vi "IV2-LCRZ.vi"(0 "Voltage In":cdb=-0.04516796338063459+0.012130821220646867i format="%#_4p", 1 "Test Frequency":dbl=25000.0, 5 "Current In":cdb=0.0013952524174977166+0.030636391761552667i format="%#_4p", 12 "LCR Params":T2={"Rg_Vmon"=5000.0, "Rg_Imon"=5000.0, "ESL_Cal"=2.95e-07, "ESR_Cal"=0.0, "Cp_Cal"=0.0, "Rp_Cal"=1000000000.0, "Use Open/Short\nCompensation"=TRUE, "R_Shunt"=100.0}) -> (4 "Impedance (Mag)":dbl=0.0009831918388061723 format="%#_3p", 6 "Impedance (Phase)":dbl=169.4760326381836 format="%#_3p", 8 "Ls":dbl=9.665874386883538e-10 format="%#_3p", 10 "Cs":dbl=-0.029973703968004497 format="%#_3p", 14 "Impedance cluster":T3={"|Z|"=0.0009831918388061723, "Phase(Z)"=169.4760326381836, "Re(Z)"=-0.000966653166475792, "Imag(Z)"=0.00017957685718763175, "Ls"=9.665874386883538e-10, "Cs"=-0.029973703968004497, "Rp"=0.0, "Cp"=0.0}, 15 "Real (Z)":dbl=-0.000966653166475792 format="%#_3p")   [LabVIEW 2020]
panel:
  out "Z":cdb
  out "Y":cdb
  in  "Cal Cluster":T1={"ESL_Cal"=2e-07, "ESR_Cal"=0.0, "Cp_Cal"=0.0, "Rp_Cal"=1000000000.0}
  out "Current Phase\nDeg":dbl=87.39241896335173
  out "Z Phase (Pre)":dbl=77.5743267290552
  out "Z Mag (pre-correction)":dbl=152.4989366461181
  out "VGain":dbl=11.0 format="%#_3p"
  out "Detected Current\n(Measured Signal \nmagnitude)":dbl=0.030668146821675832 format="%#_3p"
  out "I_Gain":dbl=11.0 format="%#_3p"
  out "Imag(Z)":dbl=0.00017957685718763175 format="%#_3p"
  out "Voltage (mag)":dbl=0.004251690708375082 format="%#_3p"
  out "Current  (Amps)":dbl=2.7880133474250757e-05 format="%#_3p"
  out "Voltage Phase\n (deg)":dbl=164.96674569240693 format="%.2p"
  out "Detected Voltage\n(Measured Signal\nMagnitude":dbl=0.0467685977921259 format="%.2p"
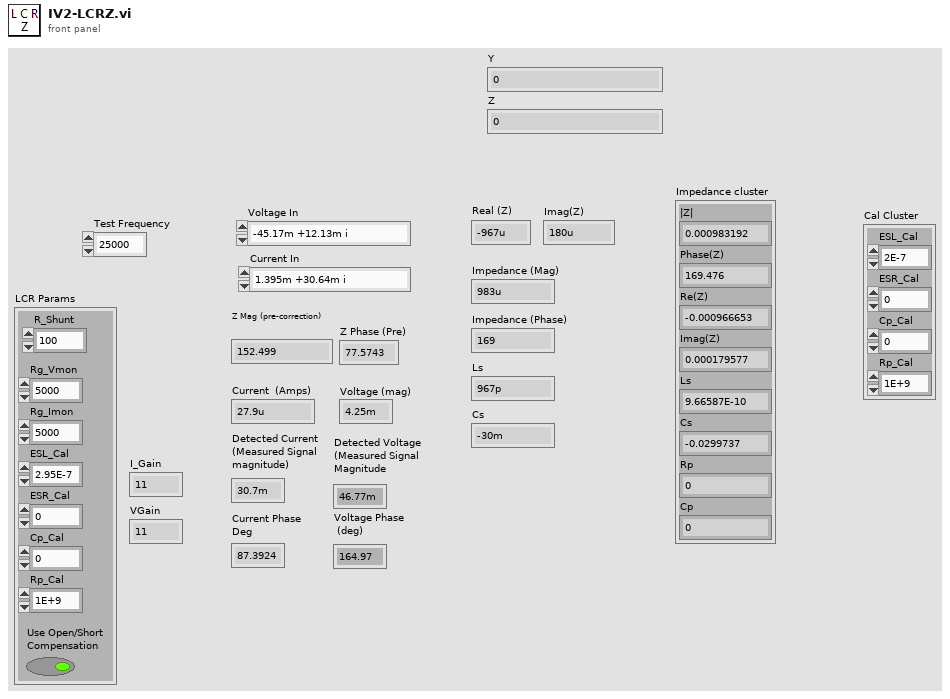
[diagram p1: front panel]
types:
  T1 = cluster{"ESL_Cal":dbl, "ESR_Cal":dbl, "Cp_Cal":dbl, "Rp_Cal":dbl}
  T2 = cluster{"Rg_Vmon":dbl, "Rg_Imon":dbl, "ESL_Cal":dbl, "ESR_Cal":dbl, "Cp_Cal":dbl, "Rp_Cal":dbl, "Use Open/Short\nCompensation":bool, "R_Shunt":dbl}
  T3 = cluster{"|Z|":dbl, "Phase(Z)":dbl, "Re(Z)":dbl, "Imag(Z)":dbl, "Ls":dbl, "Cs":dbl, "Rp":dbl, "Cp":dbl}
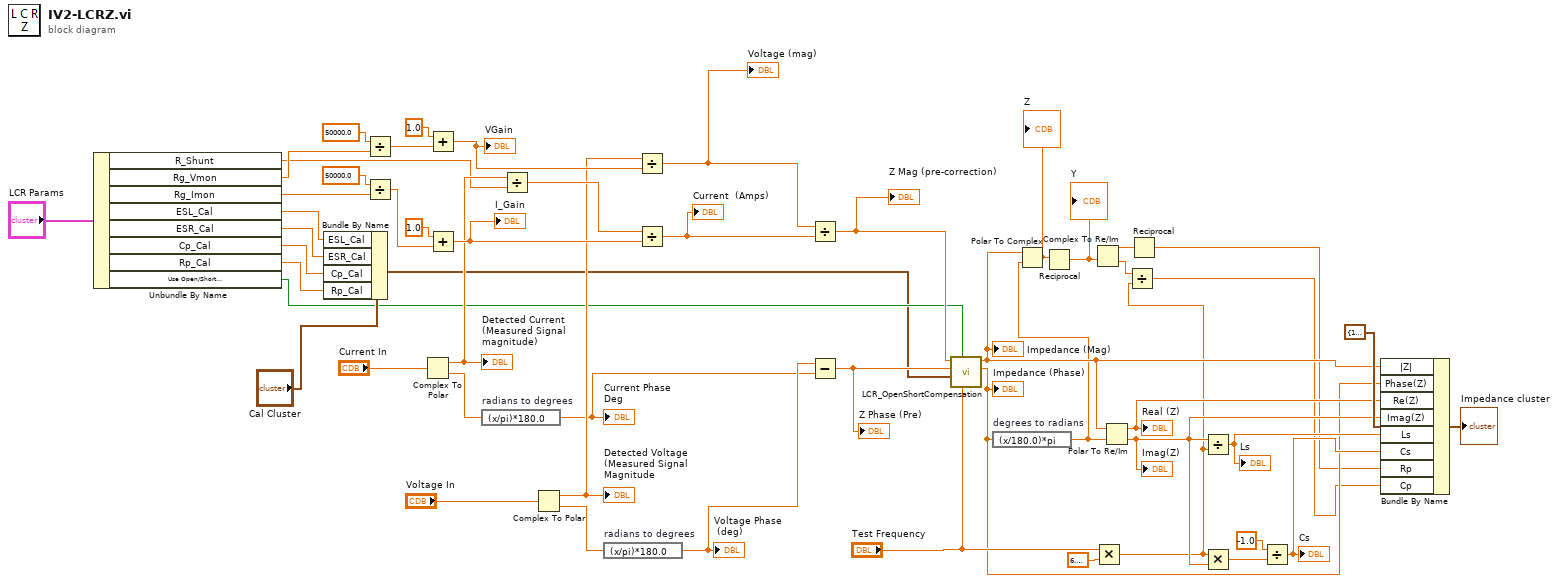
[diagram p0: block diagram]
diagram:
  n1 = Unbundle By Name("LCR Params") -> ("R_Shunt"=w12:dbl, "Rg_Vmon"=w14:dbl, "Rg_Imon"=w15:dbl, "ESL_Cal"=w19:dbl, "ESR_Cal"=w18:dbl, "Cp_Cal"=w17:dbl, "Rp_Cal"=w16:dbl, "Use Open/Short\nCompensation"=w13:bool)
  n2 = Bundle By Name(cluster="Cal Cluster", "ESL_Cal"=w19, "ESR_Cal"=w18, "Cp_Cal"=w17, "Rp_Cal"=w16) -> (w11:T1)
  n3 = Divide(x=50000.0, y=w14) -> (x/y=w44:dbl)
  n4 = Divide(x=50000.0, y=w15) -> (x/y=w48:dbl)
  n5 = Complex To Polar(r * e^(i*theta)="Current In") -> (r=w36:dbl, theta=w31:dbl)
  "Detected Current\n(Measured Signal \nmagnitude)" <- w36
  n6 = Add(x=1.0, y=w44) -> (x+y=w41:dbl)
  "VGain" <- w41
  n7 = Add(x=1.0, y=w48) -> (x+y=w46:dbl)
  "I_Gain" <- w46
  n8 = expression code="(x/pi)*180.0" "radians to degrees"(w31) -> (w30:dbl)
  "Current Phase\nDeg" <- w30
  n9 = Divide(x=w36, y=w12) -> (x/y=w47:dbl)
  n10 = Complex To Polar(r * e^(i*theta)="Voltage In") -> (r=w37:dbl, theta=w33:dbl)
  "Detected Voltage\n(Measured Signal\nMagnitude" <- w37
  n11 = expression code="(x/pi)*180.0" "radians to degrees"(w33) -> (w32:dbl)
  "Voltage Phase\n (deg)" <- w32
  n12 = Divide(x=w37, y=w41) -> (x/y=w40:dbl)
  "Voltage (mag)" <- w40
  n13 = Divide(x=w47, y=w46) -> (x/y=w45:dbl)
  "Current  (Amps)" <- w45
  n14 = Divide(x=w40, y=w45) -> (x/y=w38:dbl)
  "Z Mag (pre-correction)" <- w38
  n15 = Subtract(x=w32, y=w30) -> (x-y=w39:dbl)
  "Z Phase (Pre)" <- w39
  n16 = call "LCR_OpenShortCompensation.vi"("Freq"="Test Frequency", "UseCorrection"=w13, "Cal Cluster"=w11, "Phase Z Meas Deg"=w39, "Mag Z Meas"=w38) -> ("Phase Z DUT"=w9:dbl, "Mag Z DUT"=w10:dbl)  [unwired: 4 in, 1 out]
  "Impedance (Mag)" <- w10
  "Impedance (Phase)" <- w9
  n17 = expression code="(x/180.0)*pi" "degrees to radians"(w9) -> (w1:dbl)
  n18 = Polar To Complex(1:w1, 2:w10) -> (0:w8:cdb)
  "Z" <- w8
  n19 = Reciprocal(x=w8) -> (1/x=w7:cdb)
  "Y" <- w7
  n20 = Complex To Re/Im(x + iy=w7) -> (x=w6:dbl, y=w4:dbl)
  n21 = Multiply(x="Test Frequency", y=6.283185307179586) -> (x*y=w3:dbl)
  n22 = Polar To Re/Im(2:w1, 3:w10) -> (0:w25:dbl, 1:w26:dbl)
  "Imag(Z)" <- w25
  "Real (Z)" <- w26
  n23 = Divide(x=w4, y=w3) -> (x/y=w2:dbl)
  n24 = Reciprocal(x=w6) -> (1/x=w5:dbl)
  n25 = Divide(x=w25, y=w3) -> (x/y=w24:dbl)
  "Ls" <- w24
  n26 = Multiply(x=w3, y=w25) -> (x*y=w52:dbl)
  n27 = Divide(x=-1.0, y=w52) -> (x/y=w23:dbl)
  "Cs" <- w23
  n28 = Bundle By Name(cluster=T3 {"|Z|"=1.0, "Phase(Z)"=0.0, "Re(Z)"=1.0, "Imag(Z)"=0.0, "Ls"=1.0, "Cs"=1.0, "Rp"=1.0, "Cp"=1.0}, "|Z|"=w10, "Phase(Z)"=w9, "Re(Z)"=w26, "Imag(Z)"=w25, "Ls"=w24, "Cs"=w23, "Rp"=w5, "Cp"=w2) -> (→"Impedance cluster":T3)
